vi "Set Output Mode.vi"(8 "error in (no error)":errorcluster, 10 "Output Mode (0: Standby)":u32(ring) items=["Standby", "Operate"], 11 "VISA resource name":refnum<visa-resource-name>) -> (0 "error out":errorcluster, 3 "VISA resource name out":refnum<visa-resource-name>)   [LabVIEW 2019, in "Fluke 5XXX Series Multicalibrators.lvlib"]
doc: "This VI activates Calibrator output if it is in standby mode and deactivates it if it is in operate mode.\n\nWhen the OPERATE annunciator is lit and OPR is displayed, the output value and function shown on the Output Display is active at the selected terminals. When STBY is displayed in the Output Display, all calibrator outputs are open-circuited except for the front panel thermocouple (TC) terminals."
uses:
  Fluke 5XXX Series Multicalibrators.lvlib
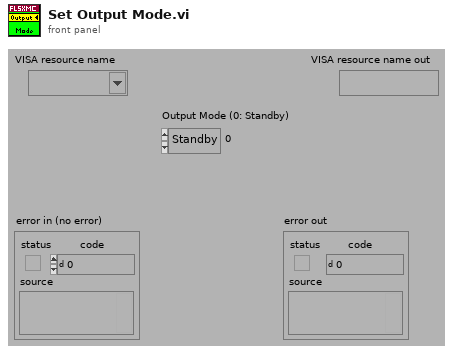
[diagram p1: front panel]
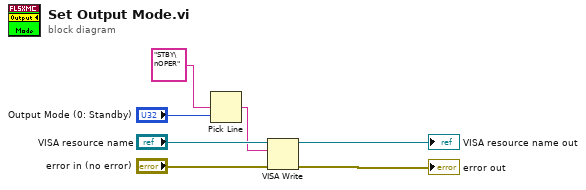
[diagram p0: block diagram]
diagram:
  n1 = Pick Line(multi-line string="STBY\nOPER" ("Reset Command"), line index="Output Mode (0: Standby)") -> (output string=w3:string)  [unwired: 1 in]
  n2 = VISA Write(VISA resource name="VISA resource name", write buffer=w3, error in (no error)="error in (no error)") -> (VISA resource name out=→"VISA resource name out":refnum<visa-resource-name>, error out=→"error out":errorcluster)  [unwired: 1 out]
